vi "LEBITplc.SetValueInRange.vi"(0 "i ref in":refnum<vi>, 1 "CommandName in":string, 2 "i attribute in":T1, 3 "value in":dbl, 4 "index of element":i32, 5 "error out in":errorcluster) -> (14 "i ref out":refnum<vi>, 15 "CommandName out":string, 17 "value out":dbl, 18 "In Range?":bool, 19 "error out":errorcluster)   [LabVIEW 2014, in "LEBITplc.lvlib"]
uses:
  LEBITplc.lvlib
  LEBITplc.i attribute.ctl
panel:
  out "Out of Range Set Value":i32
  out "i attribute out":T1
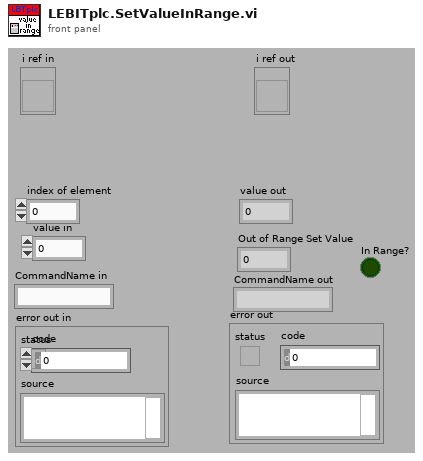
[diagram p1: front panel]
types:
  T1 = typedef "LEBITplc.lvlib/LEBITplc.i attribute.ctl" = cluster{"LLFLocation":string, "SetFileLocation":string, "nickNames":string[], "setValuePLCServiceID":i32[], "GUIServiceID":i32[], "monValuePLC":string[], "SetValueServiceID":i32[], "MonValueServiceID":i32[], "SetValue":dbl[][], "SetValueMin":dbl[], "SetValueMax":dbl[], "SetValueInfoServiceID":i32[], "GUINames":string[], "ListOfBases":string[], "Scale":dbl[], "Offset":dbl[], "setValuePLC":string[], "BaseName":string[], "ScaleServiceID":i32[], "OffsetServiceID":i32[], "AllPLCValues":string[], "CondSpecialArray":string[][], "CondSpecialIndex":i32[], "CondSpecialMonValue":dbl[], "RecentlyChanged":i32[], "SetFileLocationID":i32, "Dependent-Monitors":string[][], "LastLoadedFiles":string[], "IonGuideCalibLocation":string, "Monitor Dependent":string[], "Special":string[], "PLC?":bool[], "Start Date":string, "ListOfBasesServiceID":i32, "SETRA VISA resource":refnum<visa-resource-name>}
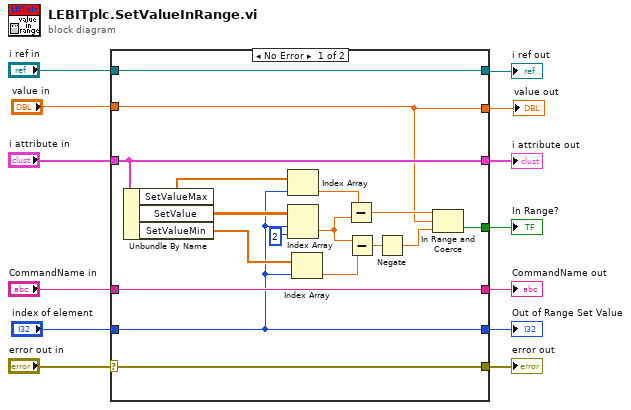
[diagram p0: block diagram]
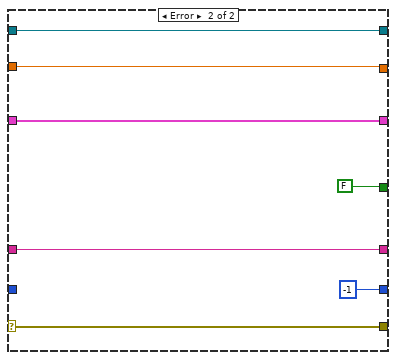
[diagram p2: hidden frame]
diagram:
  n1 = case shown="No Error" "error out in" {
    selector: "error out in" -> [w30 w35]
    tunnel: "i ref in" -> [w29 w37]
    tunnel: "i attribute in" -> [w28 w36]
    tunnel: [w29 w37] -> w9
    tunnel: [w30 w35] -> w10
    tunnel: [w28 w36] -> w8
    tunnel: "CommandName in" -> [w26 w33]
    tunnel: [w21 FALSE] -> w6
    tunnel: [w26 w33] -> w5
    tunnel: [w14 -1 ("index of element")] -> w4
    tunnel: "value in" -> [w16 w31]
    tunnel: [w16 w31] -> w2
    tunnel: "index of element" -> [w14 _]
    frame No Error {
      n2 = Unbundle By Name(w28) -> ("SetValueMax"=w19:dbl[], "SetValue"=w27:dbl[][], "SetValueMin"=w18:dbl[])
      n3 = Index Array(array=w19, index=w14) -> (element=w20:dbl)
      n4 = Index Array(array=w27, index (row)=w14, index (col)=2 ("index")) -> (element=w25:dbl)
      n5 = Index Array(array=w18, index=w14) -> (element=w17:dbl)
      n6 = Subtract(x=w20, y=w25) -> (x-y=w24:dbl)
      n7 = Subtract(x=w25, y=w17) -> (x-y=w23:dbl)
      n8 = Negate(x=w23) -> (-x=w22:dbl)
      n9 = In Range and Coerce(upper limit=w24, x=w16, lower limit=w22) -> (In Range?=w21:bool)  [unwired: 1 out]
    }
    frame Error {
    }
  }
  "error out" <- w10
  "i attribute out" <- w8
  "i ref out" <- w9
  "In Range?" <- w6
  "CommandName out" <- w5
  "Out of Range Set Value" <- w4
  "value out" <- w2
